vi "LoadConfig_Dash.vi"(10 "ControlsToLoad":refnum<vi>[](array[refnum]), 11 "Path":path) -> ()   [LabVIEW 2015]
uses:
  <vilib>/Utility/config.llb/NI_LVConfig.lvlib
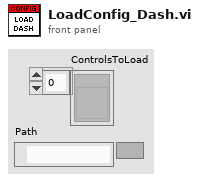
[diagram p1: front panel]
types:
  T1 = typedef "NI_LVConfig.lvlib/Config Data RefNum.ctl" = refnum<k1>
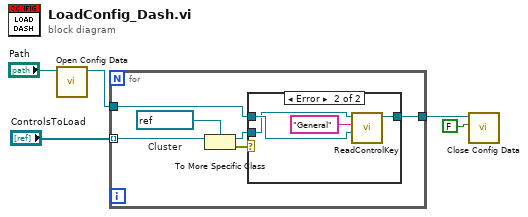
[diagram p0: block diagram]
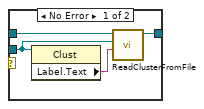
[diagram p2: hidden frame]
diagram:
  n1 = call <vilib>:"Open Config Data.vi"("configuration file path"="Path") -> ("refnum"=w3:T1)  [unwired: 8 in, 2 out]
  n2 = for {
    tunnel: "ControlsToLoad" -> [w11] mode=indexing
    tunnel: w3 -> [w8]
    tunnel: [w6] -> w2
    w10 = refnum<vi> refnum  # Cluster
    n3 = To More Specific Class(target class=w10, reference=w11) -> (specific class reference=w7:refnum<vi>, error out=w9:errorcluster)  [unwired: 1 in]
    n4 = case shown="Error" w9 {
      tunnel: w8 -> [w15 w19]
      tunnel: w7 -> [w14 w18]
      tunnel: [w12 w16] -> w6
      frame No Error {
        n5 = property class="Clust"(reference=w14) -> ("Label.Text"=w13:string)  [unwired: 1 in, 2 out]
        n6 = call "ReadClusterFromFile.vi"("Name"=w13, "Cluster in"=w14, "ConfigIn"=w15) -> ("ConfigOut"=w12:T1)  [unwired: 8 in]
      }
      frame Error {
        n7 = call "ReadControlKey.vi"("ConfigFile"=w19, "section"="General", "Control in"=w18) -> ("ConfigFile out"=w16:T1)  [unwired: 8 in]
      }
    }
  }
  n8 = call <vilib>:"Close Config Data.vi"("write file if changed (T)"=FALSE, "refnum"=w2) -> ()  [unwired: 8 in, 2 out]
